vi "Set Drive Outputs.vi"(0 "Front Left":dbl, 1 "Inv Front Left":bool, 2 "Front Right":dbl, 3 "Inv Front Right":bool, 4 "Rear Left":dbl, 5 "Inv Rear Left":bool, 6 "Rear Right":dbl, 7 "Inv Rear Right":bool) -> ()   [LabVIEW 2012]
uses:
  Globals/Jaguar Commands.vi
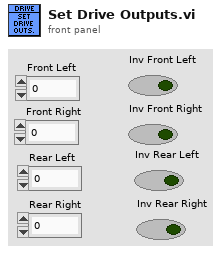
[diagram p1: front panel]
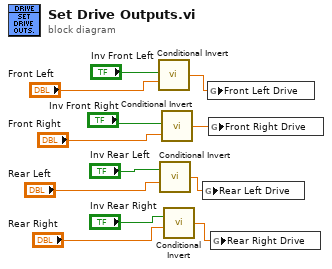
[diagram p0: block diagram]
diagram:
  n1 = call "Conditional Invert.vi"("x"="Front Left", "invert"="Inv Front Left") -> ("invert ? x : -x"=w10:dbl)  [unwired: 1 in]
  n2 = call "Conditional Invert.vi"("x"="Rear Left", "invert"="Inv Rear Left") -> ("invert ? x : -x"=w4:dbl)  [unwired: 1 in]
  n3 = call "Conditional Invert.vi"("x"="Front Right", "invert"="Inv Front Right") -> ("invert ? x : -x"=w8:dbl)  [unwired: 1 in]
  n4 = call "Conditional Invert.vi"("x"="Rear Right", "invert"="Inv Rear Right") -> ("invert ? x : -x"=w1:dbl)  [unwired: 1 in]
  n5 = global write "Jaguar Commands.vi" "Rear Left Drive"(w4) -> ()
  n6 = global write "Jaguar Commands.vi" "Front Left Drive"(w10) -> ()
  n7 = global write "Jaguar Commands.vi" "Front Right Drive"(w8) -> ()
  n8 = global write "Jaguar Commands.vi" "Rear Right Drive"(w1) -> ()
